vi "execute.vi"(8 "error in (no error)":errorcluster, 9 "image assembler in":refnum<class "GenericComponent.lvclass">, 10 "imaging mode in":refnum<class "GenericComponent.lvclass">, 11 "adapter in":refnum<class "AdapterMG090625ImagingModeToImageAssembler.lvclass">) -> (0 "error out":errorcluster, 1 "image assembler out":refnum<class "GenericComponent.lvclass">, 2 "imaging mode out":refnum<class "GenericComponent.lvclass">, 3 "adapter out":refnum<class "AdapterMG090625ImagingModeToImageAssembler.lvclass">)   [LabVIEW 2010, in "AdapterMG090625ImagingModeToImageAssembler.lvclass"]
uses:
  AdapterMG090625ImagingModeToImageAssembler.lvclass
  common/classes/GenericComponent/GenericComponent/GenericComponent.lvclass
  ImageAssembler/ImageAssemblerMG090623Binning/ImageAssemblerMG090623Binning/ImageAssemblerMG090623Binning.lvclass
  ImagingMode/ImagingModeMG090624Camera/ImagingModeMG090624Camera/ImagingModeMG090624Camera.lvclass
panel:
  # "imaging mode: ImagingModeMG090624Camera\nimage assembler: ImageAssemblerMG090623Binning"
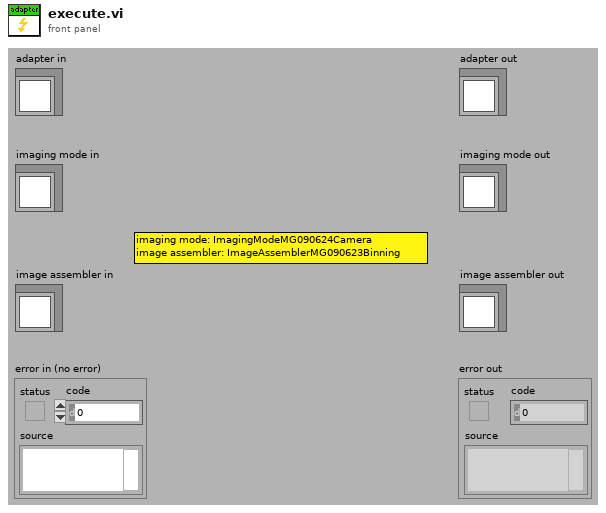
[diagram p1: front panel]
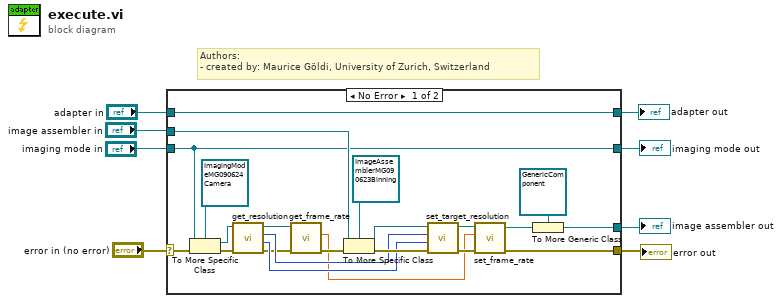
[diagram p0: block diagram]
diagram:
  # "Authors: \n- created by: Maurice Göldi, University of Zurich, Switzerland"
  n1 = case shown="No Error" "error in (no error)" {
    selector: "error in (no error)" -> [w29 w34]
    tunnel: [w17 w34] -> w6
    tunnel: [w27 w33] -> w7
    tunnel: "adapter in" -> [w27 w33]
    tunnel: "imaging mode in" -> [w25 w31]
    tunnel: "image assembler in" -> [w28 w32]
    tunnel: [w26 w32] -> w1
    tunnel: [w25 w31] -> w2
    frame No Error {
      n2 = To More Specific Class(target class=refnum<class "ImagingModeMG090624Camera.lvclass"> refnum ("ImagingModeMG090624Camera.lvclass"), reference=w25, error in=w29) -> (specific class reference=w23:refnum<class "ImagingModeMG090624Camera.lvclass">, error out=w24:errorcluster)
      n3 = call-dynamic "get_resolution.vi"("error in (no error)"=w24, "ScanModeMG090624Camera in"=w23) -> ("error out"=w14:errorcluster, "y"=w19:i32, "x"=w20:i32, "ScanModeMG090624Camera out"=w12:refnum<class "ImagingModeMG090624Camera.lvclass">)  [unwired: 6 in]
      n4 = call-dynamic "get_frame_rate.vi"("error in (no error)"=w14, "ScanModeMG090624Camera in"=w12) -> ("error out"=w13:errorcluster, "frame rate"=w11:dbl[unit])  [unwired: 8 out]
      n5 = To More Specific Class(target class=refnum<class "ImageAssemblerMG090623Binning.lvclass"> refnum ("ImageAssemblerMG090623Binning.lvclass"), reference=w28, error in=w13) -> (specific class reference=w21:refnum<class "ImageAssemblerMG090623Binning.lvclass">, error out=w22:errorcluster)
      n6 = call-dynamic "set_target_resolution.vi"("error in (no error)"=w22, "y"=w19, "x"=w20, "MG090623BinningImageAssembler.lvclass in"=w21) -> ("error out"=w18:errorcluster, "MG090623BinningImageAssembler.lvclass out"=w16:refnum<class "ImageAssemblerMG090623Binning.lvclass">)  [unwired: 6 in]
      n7 = call-dynamic "set_frame_rate.vi"("error in (no error)"=w18, "frame rate"=w11, "MG090623BinningImageAssembler.lvclass in"=w16) -> ("error out"=w17:errorcluster, "MG090623BinningImageAssembler.lvclass out"=w15:refnum<class "ImageAssemblerMG090623Binning.lvclass">)  [unwired: 7 out]
      n8 = To More Generic Class(target class=refnum<class "GenericComponent.lvclass"> refnum ("GenericComponent.lvclass"), reference=w15) -> (generic class reference=w26:refnum<class "GenericComponent.lvclass">)
    }
    frame Error {
    }
  }
  "error out" <- w6
  "adapter out" <- w7
  "imaging mode out" <- w2
  "image assembler out" <- w1
